vi "Create Filled Text Fields.vi"(8 "error in (no error)":errorcluster, 11 "Filled Text Fields Ref":refnum<vi>) -> (0 "error out":errorcluster, 3 "Filled Text Fields Reference":refnum<class "Message Enqueuer.lvclass">)   [LabVIEW 2017, in "Filled Text Fields.lvlib" / "Filled Text Fields Actor.lvclass"]
uses:
  Filled Text Fields Actor.lvclass
  <vilib>/ActorFramework/Message Enqueuer/Message Enqueuer.lvclass
  C:/Program Files (x86)/National Instruments/LabVIEW 2017/vi.lib/ActorFramework/Actor/Actor.lvclass
  Filled Text Fields Actor.lvclass/Filled Text Fields Actor.ctl
  <vilib>/ActorFramework/Actor/Actor.lvclass
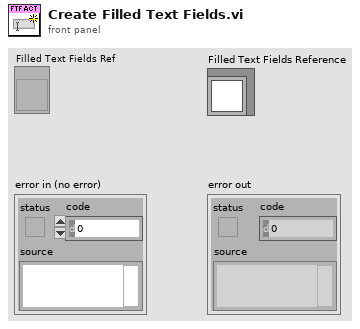
[diagram p1: front panel]
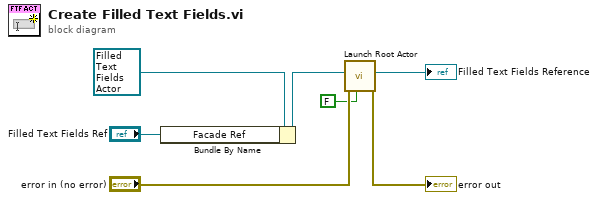
[diagram p0: block diagram]
diagram:
  n1 = Bundle By Name(cluster=refnum<class "Filled Text Fields Actor.lvclass"> refnum ("Filled Text Fields Actor in"), "Facade Ref"="Filled Text Fields Ref") -> (w3:refnum<class "Filled Text Fields Actor.lvclass">)
  n2 = call <vilib>:"Launch Root Actor.vi"("Open Actor Core front panel? (F)"=FALSE, "error in (no error)"="error in (no error)", "Actor"=w3) -> ("error out"=→"error out":errorcluster, "Actor's Enqueuer"=→"Filled Text Fields Reference":refnum<class "Message Enqueuer.lvclass">)  [unwired: 7 in]
